vi "TimeCardStorage.vi"(2 "error in (no error)":errorcluster, 3 "Timing Card Settings":T1[](array[typedef]), 4 "Timing Channel Settings":T2[][](array[typedef]) {"FrontPanelTime" format="%.3p"; "Pulse width (s)" format="%.3p"; "Delay (s)" format="%.3p"}, 5 "Data Value Reference in":refnum<data-value>) -> (0 "error out":errorcluster)   [LabVIEW 2014]
uses:
  <vilib>/MDSplus/Classes/Tree_Class/Tree.lvclass
  Controls/TimingChannelSettings.ctl
  Controls/TimingCardSettings.ctl
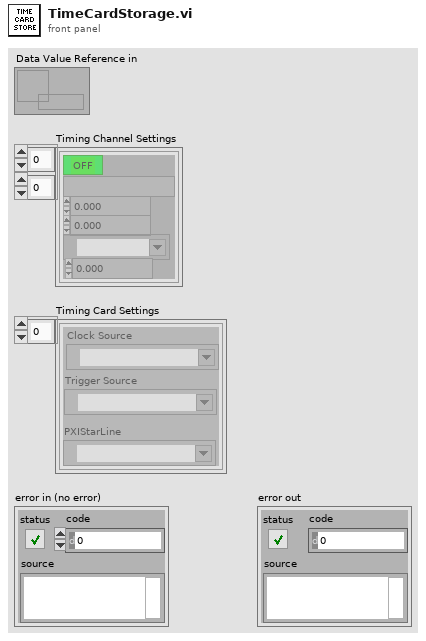
[diagram p1: front panel]
types:
  T1 = typedef "TimingCardSettings.ctl" = cluster{"Trigger Source":tag, "Clock Source":tag, "PXIStarLine":tag}
  T2 = typedef "TimingChannelSettings.ctl" = cluster{"Delay (s)":dbl, "Pulse width (s)":dbl, "Active":bool, "Channel Name":string, "counter":tag, "FrontPanelTime":dbl}
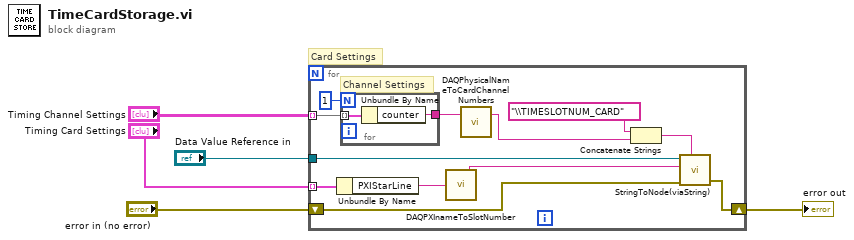
[diagram p0: block diagram]
diagram:
  # "Card Settings"
  n1 = for {
    tunnel: "Data Value Reference in" -> [w15]
    shift-right: [w13] -> w1
    shift-left: "error in (no error)" -> [w14]
    tunnel: "Timing Card Settings" -> [w17] mode=indexing
    tunnel: "Timing Channel Settings" -> [w9] mode=indexing
    # "Channel Settings"
    n2 = Unbundle By Name(w17) -> ("PXIStarLine"=w11:tag)
    n3 = for {
      N: 1 -> [_]
      tunnel: w9 -> [w19] mode=indexing
      tunnel: [w18] -> w12
      n4 = Unbundle By Name(w19) -> ("counter"=w18:tag)
    }
    n5 = call "DAQPXInameToSlotNumber.vi"("PXI name"=w11) -> ("Slot #"=w10:string)
    n6 = call "DAQPhysicalNameToCardChannelNumbers.vi"("NI Physical Channel"=w12) -> ("Card #"=w8:string)  [unwired: 1 in, 1 out]
    n7 = Concatenate Strings("\\TIMESLOTNUM_CARD" ("string"), w8) -> (w16:string)
    n8 = call "StringToNode(viaString).vi"("Tree DVR in"=w15, "String value in"=w10, "error in (no error)"=w14, "NodePath"=w16) -> ("error out"=w13:errorcluster)  [unwired: 2 in, 1 out]
  }
  "error out" <- w1
